vi "Read instrument handle.vi"(8 "error in (no error)":errorcluster, 11 "Thorlabs_PM100D in":refnum<class "Thorlabs_PM100D.lvclass">) -> (0 "error out":errorcluster, 2 "instrument handle":refnum<visa-resource-name>, 3 "Thorlabs_PM100D out":refnum<class "Thorlabs_PM100D.lvclass">)   [LabVIEW 2020, in "Thorlabs_PM100D.lvclass"]
uses:
  <instrlib>/Classes/Powermeter/Thorlabs_PM100D/Thorlabs_PM100D.lvclass
  <instrlib>/Classes/Powermeter/Thorlabs_PM100D/Thorlabs_PM100D.lvclass/Thorlabs_PM100D.ctl
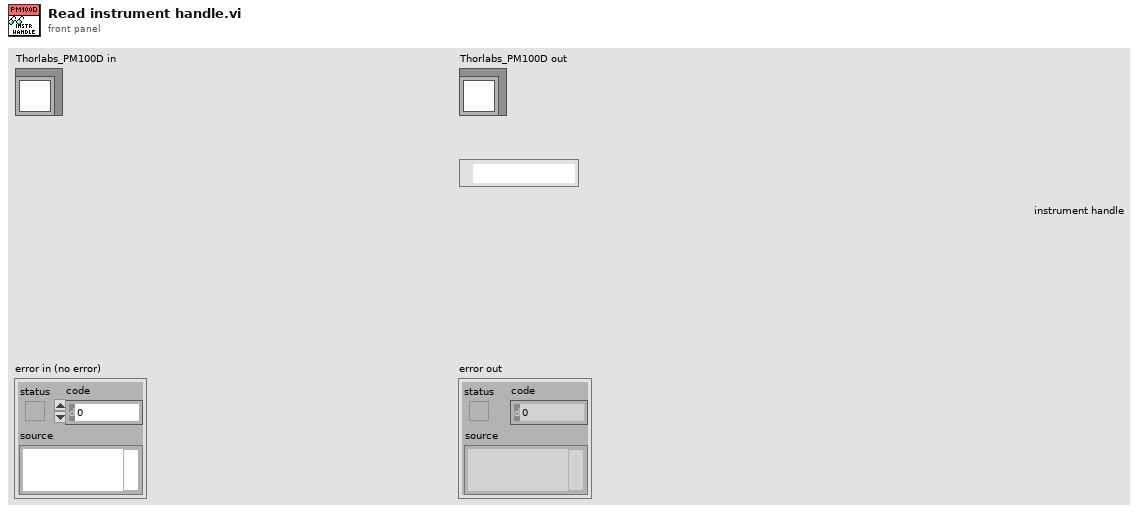
[diagram p1: front panel]
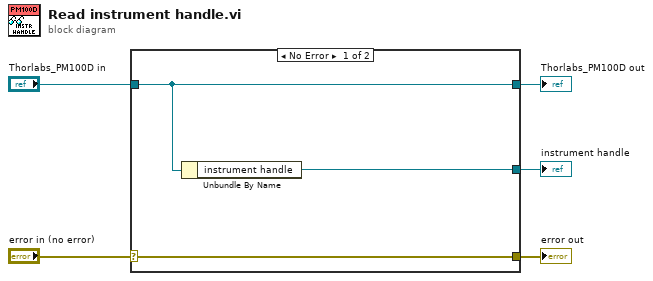
[diagram p0: block diagram]
diagram:
  n1 = case shown="No Error" "error in (no error)" {
    selector: "error in (no error)" -> [w8 w9]
    tunnel: [w8 w9] -> w4
    tunnel: [w7 w10] -> w2
    tunnel: "Thorlabs_PM100D in" -> [w7 w10]
    tunnel: [w6 _] -> w1
    frame No Error {
      n2 = Unbundle By Name(w7) -> ("instrument handle"=w6:refnum<visa-resource-name>)
    }
    frame Error {
    }
  }
  "error out" <- w4
  "Thorlabs_PM100D out" <- w2
  "instrument handle" <- w1
